vi "2comp2dec.vi"(2 "factor":dbl=1.0, 3 "two' complement":u16=6553) -> (0 "decimal":dbl)   [LabVIEW 2021]
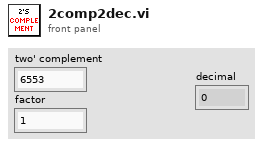
[diagram p1: front panel]
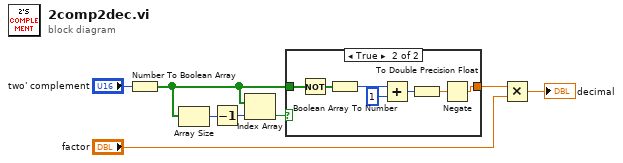
[diagram p0: block diagram]
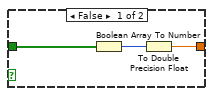
[diagram p2: hidden frame]
diagram:
  n1 = Number To Boolean Array(number="two' complement") -> (Boolean array=w3:bool[])
  n2 = Array Size(array=w3) -> (size(s)=w2:i32)
  n3 = Decrement(x=w2) -> (x-1=w1:i32)
  n4 = Index Array(array=w3, index=w1) -> (element=w8:bool)
  n5 = case shown="True" w8 {
    tunnel: w3 -> [w11 w18]
    tunnel: [w10 w14] -> w6
    frame False {
      n6 = Boolean Array To Number(Boolean array=w11) -> (number=w9:u32)
      n7 = To Double Precision Float(number=w9) -> (double precision float=w10:dbl)
    }
    frame True {
      n8 = Not(x=w18) -> (.not. x?=w15:bool[])
      n9 = Boolean Array To Number(Boolean array=w15) -> (number=w17:u32)
      n10 = Add(x=w17, y=u32 1) -> (x+y=w13:u32)
      n11 = To Double Precision Float(number=w13) -> (double precision float=w12:dbl)
      n12 = Negate(x=w12) -> (-x=w14:dbl)
    }
  }
  n13 = Multiply(x=w6, y="factor") -> (x*y=→"decimal":dbl)
